vi "Filter.vi"(8 "error in (no error)":errorcluster, 10 "Selected Runnables":string[](array[string]), 11 "LUnit Test Suite V2 In":refnum<class "LUnit Test Suite V2.lvclass">) -> (0 "error out":errorcluster, 3 "LUnit Test Suite V2 Out":refnum<class "LUnit Test Suite V2.lvclass">)   [LabVIEW 2020, in "LUnit Test Suite V2.lvclass"]
uses:
  LUnit Test Suite V2.lvclass
  LUnit Test Suite V2.lvclass/LUnit Test Suite V2.ctl
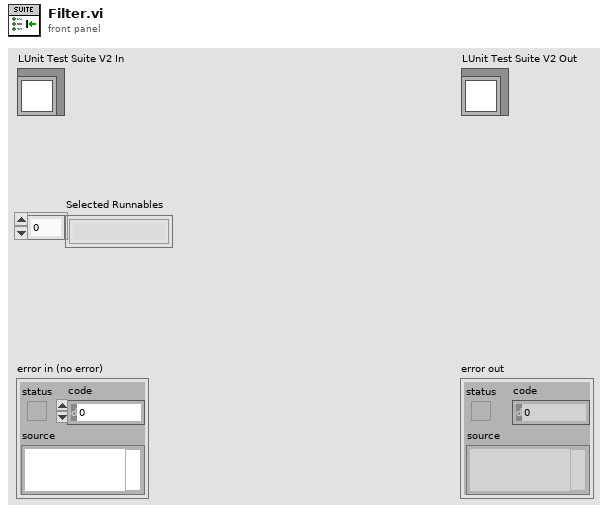
[diagram p1: front panel]
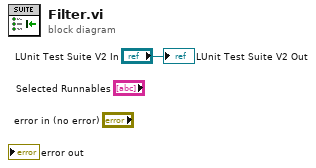
[diagram p0: block diagram]
diagram:
  "LUnit Test Suite V2 Out" <- "LUnit Test Suite V2 In"
